vi "TestExec.Config, Get Released SW List.vi"(11 "Path":path=path "C:/MTE/Test Executive/Config") -> (0 "error out":errorcluster, 2 "SW List Array":string[][](array[string]), 3 "SW List":variant)   [LabVIEW 2018]
uses:
  <vilib>/Utility/config.llb/Read Key (String).vi
  <vilib>/Utility/config.llb/NI_LVConfig.lvlib
  <vilib>/KATE/Files/File Utils.lvlib
  <vilib>/KATE/Strings/String Utils.lvlib
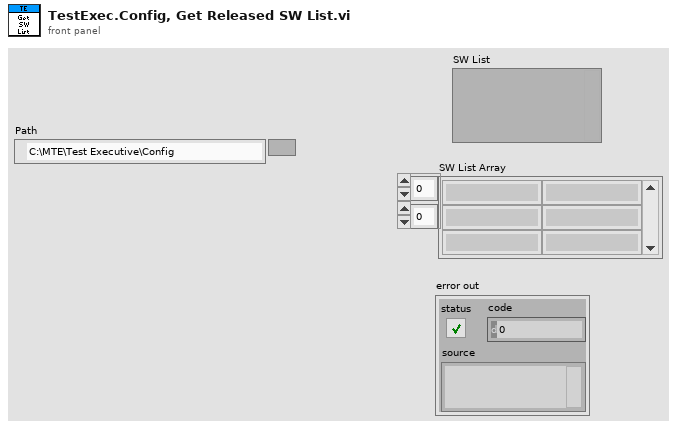
[diagram p1: front panel]
types:
  T1 = typedef "NI_LVConfig.lvlib/Config Data RefNum.ctl" = refnum<k1>
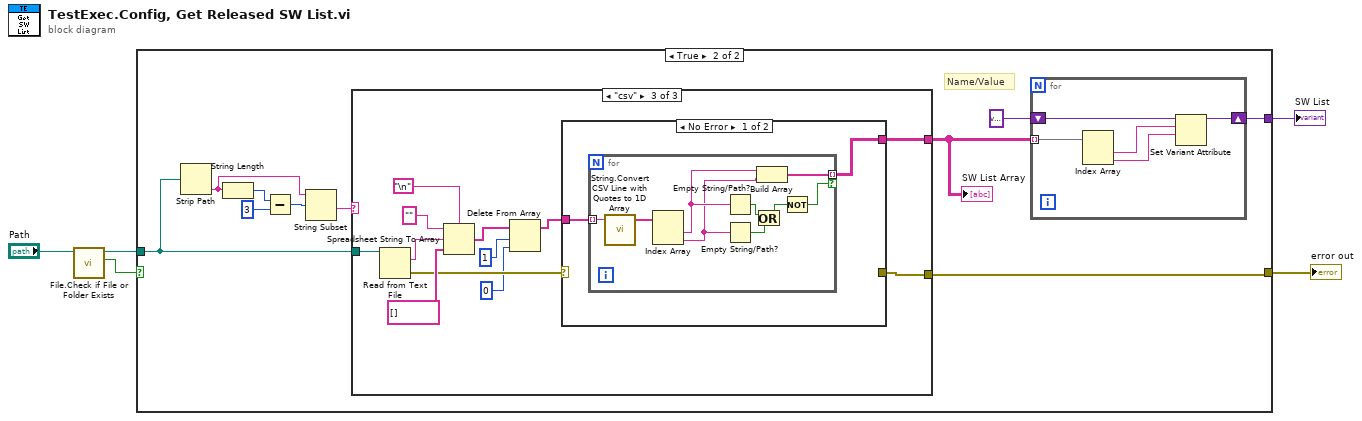
[diagram p0: block diagram]
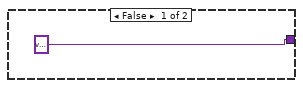
[diagram p2: hidden frame]
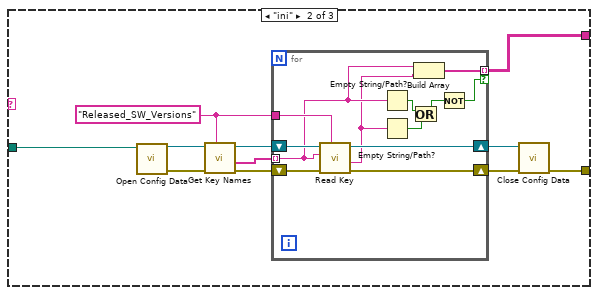
[diagram p4: hidden frame]
diagram:
  n1 = call <vilib>:"File.Check if File or Folder Exists.vi"("Path"="Path") -> ("Exists"=w1:bool, "Dup Path"=w2:path)  [unwired: 6 in, 3 out]
  n2 = case shown="True" w1 {
    tunnel: [_ w16] -> w5
    tunnel: w2 -> [_ w7]
    tunnel: [variant w14] -> w3
    frame False {
    }
    frame True {
      # "Name/Value"
      n3 = Strip Path(path=w7) -> (name=w9:string)  [unwired: 1 out]
      n4 = String Length(string=w9) -> (length=w11:i32)
      n5 = Subtract(x=w11, y=3) -> (x-y=w12:i32)
      n6 = String Subset(string=w9, offset (0)=w12) -> (substring=w8:string)  [unwired: 1 in]
      n7 = case shown="\"csv\"" w8 {
        tunnel: w7 -> [_ w27 w50]
        tunnel: [_ w19 w44] -> w16
        tunnel: [_ w18 w51] -> w13
        frame Default {
          # "Do Nothing"
        }
        frame "ini" {
          w26 = "Released_SW_Versions" ("section")
          n8 = call <vilib>:"Open Config Data.vi"("configuration file path"=w27) -> ("error out"=w17:errorcluster, "refnum"=w25:T1)  [unwired: 8 in, 1 out]
          n9 = call <vilib>:"Get Key Names.vi"("section"=w26, "error in (no error)"=w17, "refnum"=w25) -> ("error out"=w22:errorcluster, "key names"=w21:string[], "refnum out"=w24:T1)  [unwired: 5 in, 1 out]
          n10 = for {
            tunnel: w26 -> [w39]
            shift-right: [w37] -> w23
            shift-left: w24 -> [w38]
            shift-right: [w36] -> w20
            shift-left: w22 -> [w35]
            tunnel: w21 -> [w32] mode=indexing
            tunnel: [w34] -> w18 mode=indexing if=w33
            n11 = call-poly <vilib>:"Read Key.vi"("section"=w39, "error in (no error)"=w35, "key"=w32, "refnum"=w38) -> ("error out"=w36:errorcluster, "value"=w31:string, "refnum out"=w37:T1)  [unwired: 4 in, 1 out]
            n12 = Empty String/Path?(string/path=w32) -> (empty?=w29:bool)
            n13 = Empty String/Path?(string/path=w31) -> (empty?=w30:bool)
            n14 = Or(x=w29, y=w30) -> (x .or. y?=w28:bool)
            n15 = Build Array(w32, w31) -> (w34:string[])
            n16 = Not(x=w28) -> (.not. x?=w33:bool)
          }
          n17 = call <vilib>:"Close Config Data.vi"("error in (no error)"=w20, "refnum"=w23) -> ("error out"=w19:errorcluster)  [unwired: 8 in, 1 out]
        }
        frame "csv" {
          n18 = Read from Text File(file (use dialog)=w50) -> (text=w49:string, error out=w45:errorcluster)  [unwired: 3 in, 2 out]
          n19 = Spreadsheet String To Array(delimiter (Tab)="\n", format string="", spreadsheet string=w49, array type (2D Dbl)=string[] []) -> (array=w42:string[])
          n20 = Delete From Array(array=w42, length=1, index=0 ("length")) -> (array with subset deleted=w43:string[])  [unwired: 1 out]
          n21 = case shown="No Error" w45 {
            selector: w45 -> [_ w63]
            tunnel: [w53 _] -> w51
            tunnel: w43 -> [w52 _]
            tunnel: [_ w63] -> w44
            frame No Error {
              n22 = for {
                tunnel: w52 -> [w57] mode=indexing
                tunnel: [w62] -> w53 mode=indexing if=w61
                n23 = call <vilib>:"String.Convert CSV Line with Quotes to 1D Array.vi"("CSV String"=w57) -> ("Array"=w56:string[])  [unwired: 9 in, 1 out]
                n24 = Index Array(array=w56) -> (element #1=w55:string, element #2=w54:string)  [unwired: 2 in]
                n25 = Empty String/Path?(string/path=w55) -> (empty?=w59:bool)
                n26 = Empty String/Path?(string/path=w54) -> (empty?=w60:bool)
                n27 = Or(x=w59, y=w60) -> (x .or. y?=w58:bool)
                n28 = Build Array(w55, w54) -> (w62:string[])
                n29 = Not(x=w58) -> (.not. x?=w61:bool)
              }
            }
            frame Error {
            }
          }
        }
      }
      "SW List Array" <- w13
      n30 = for {
        shift-right: [w67] -> w14
        shift-left: variant ("Rel_SW") -> [w68]
        tunnel: w13 -> [w66] mode=indexing
        n31 = Index Array(array=w66) -> (element #1=w64:string, element #2=w65:string)  [unwired: 2 in]
        n32 = Set Variant Attribute(Variant=w68, name=w64, value=w65) -> (Variant out=w67:variant)  [unwired: 1 in, 2 out]
      }
    }
  }
  "error out" <- w5
  "SW List" <- w3
